vi "Debug.vi"(8 "error in (no error)":errorcluster, 9 "Numeric 2":dbl, 10 "Numeric 1":dbl, 11 "Freezer in":refnum<class "Freezer.lvclass">) -> (0 "error out":errorcluster, 3 "Freezer out":refnum<class "Freezer.lvclass">)   [LabVIEW 2015, in "cRIO-Carbondioxide.lvlib" / "CO2-Actor.lvlib" / "Freezer.lvclass"]
uses:
  Freezer.lvclass
  cRIO-CO2/Debugger Graph cluster.ctl
  cRIO-CO2/cRIO-CO2.lvclass
  CO2 Actor/CO2 Actor.lvclass
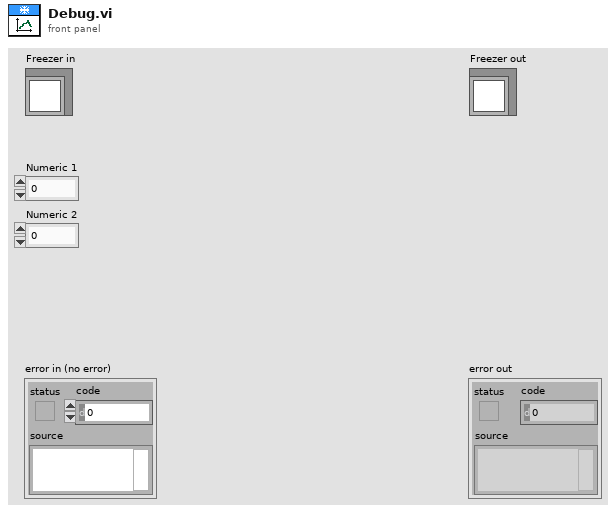
[diagram p1: front panel]
types:
  T1 = typedef "cRIO-Carbondioxide.lvlib/cRIO-CO2.lvlib/cRIO-CO2.lvclass/Debugger Graph cluster.ctl" = cluster{"Numeric 1":dbl, "Numeric 2":dbl, "Numeric 3":dbl, "Numeric 4":dbl, "Numeric 5":dbl, "Numeric 6":dbl, "Numeric 7":dbl, "Numeric 8":dbl}
  T2 = typedef "cRIO-Carbondioxide.lvlib/cRIO-CO2.lvlib/cRIO-CO2.lvclass/Debugger.ctl" = cluster{"Log Ref":refnum<vi>, "Debugger Graph Chart Ref":refnum<vi>, "Debug Rng Ref":refnum<vi>}
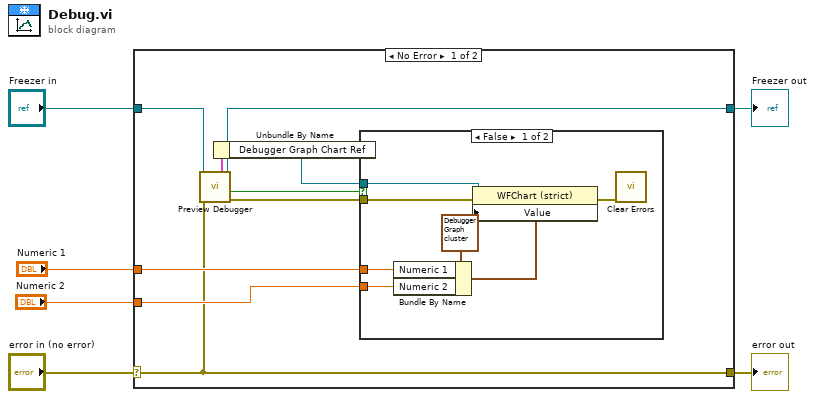
[diagram p0: block diagram]
diagram:
  n1 = case shown="No Error" "error in (no error)" {
    selector: "error in (no error)" -> [w12 w24]
    tunnel: [w12 w24] -> w5
    tunnel: [w13 w23] -> w3
    tunnel: "Freezer in" -> [w10 w23]
    tunnel: "Numeric 1" -> [w15 _]
    tunnel: "Numeric 2" -> [w14 _]
    frame No Error {
      n2 = call "Preview Debugger.vi"("error in (no error)"=w12, "CO2 Actor in"=w10) -> ("error out"=w11:errorcluster, "timed out?"=w9:bool, "Debugger"=w8:T2, "CO2 Actor out"=w13:refnum<class "Freezer.lvclass">)  [unwired: 6 in]
      n3 = Unbundle By Name(w8) -> ("Debugger Graph Chart Ref"=w7:refnum<vi>)
      n4 = case shown="False" w9 {
        tunnel: w11 -> [w21 _]
        tunnel: w7 -> [w22 _]
        tunnel: w15 -> [w20 _]
        tunnel: w14 -> [w19 _]
        frame False {
          n5 = Bundle By Name(cluster=T1 {"Numeric 1"=nan, "Numeric 2"=nan, "Numeric 3"=nan, "Numeric 4"=nan, "Numeric 5"=nan, "Numeric 6"=nan, "Numeric 7"=nan, "Numeric 8"=nan} ("Cluster"), "Numeric 1"=w20, "Numeric 2"=w19) -> (w16:T1)
          n6 = property class="WFChart (strict)"(reference=w22, error in=w21, "Value"=w16) -> (error out=w18:errorcluster)  [unwired: 1 out]
          n7 = call <vilib>:"Clear Errors.vi"("error in (no error)"=w18) -> ()  [unwired: 5 in, 2 out]
        }
        frame True {
        }
      }
    }
    frame Error {
    }
  }
  "error out" <- w5
  "Freezer out" <- w3
